vi "Write RC Parameters.vi"(0 "JSON FilePath":path=path "F:/Backup/ZenGage v3.0/20-02-2018/ZenGage v1.1/Configuration file/Rack Controller JSON/Rack Controller Override JSON.json", 1 "Part Name":string="102", 2 "RC parameters variant":variant, 5 "M and N array":T2(array[cluster])=[{"M1"=1, "M2"=2, "N1"=3, "N2"=4}, {"M1"=5, "M2"=6, "N1"=7, "N2"=8}, {"M1"=9, "M2"=10, "N1"=11, "N2"=12}], 7 "Enabled Disable Array":bool[](array[boolean]), 9 "Ticked measurements":i32[](array[numeric])=[0, 2, 4], 11 "error in (no error)":errorcluster, 12 "Rack Id":string="0", 13 "Variant":bool) -> (4 "JSON Variant":variant, 15 "error out":errorcluster)   [LabVIEW 2019, in "ZenGage v3.0 UI.lvclass"]
uses:
  ZenGage v3.0 UI.lvclass
panel:
  out "data":T1
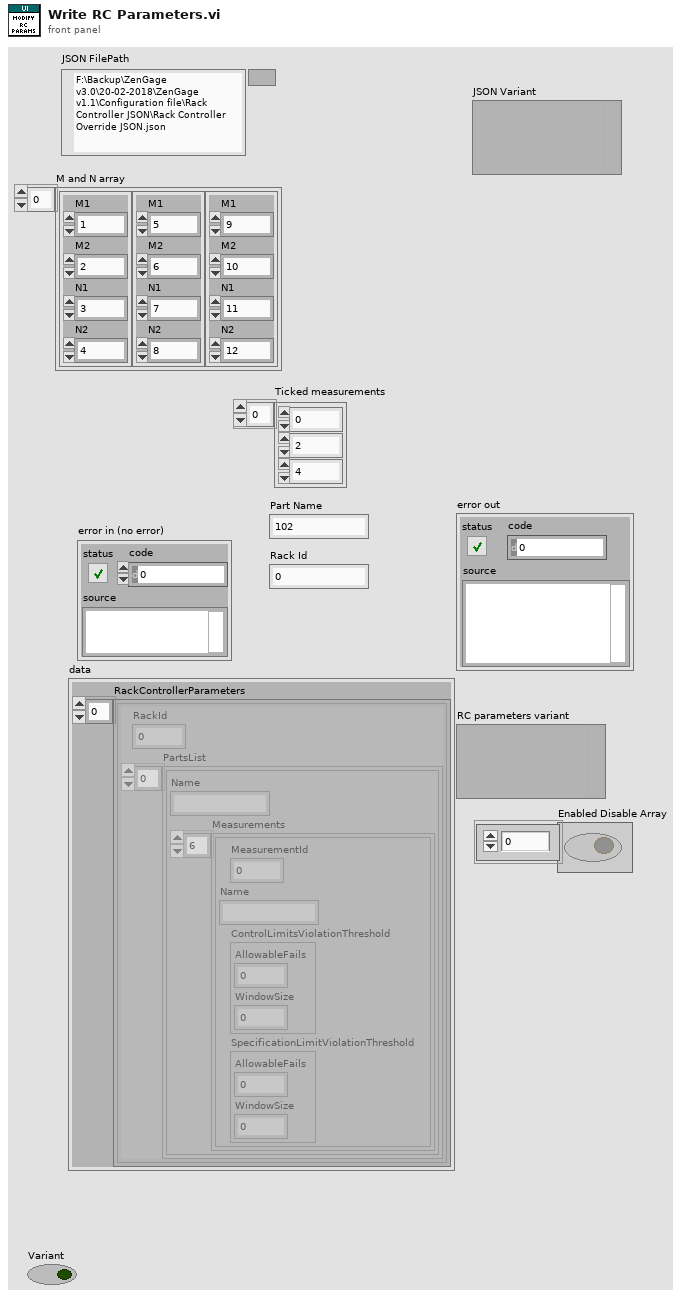
[diagram p1: front panel]
types:
  T1 = cluster{"RackControllerParameters":cluster{"RackId":dbl, "PartsList":cluster{"Name":string, "Measurements":cluster{"MeasurementId":dbl, "Name":string, "ControlLimitsViolationThreshold":cluster{"AllowableFails":dbl, "WindowSize":dbl}, "SpecificationLimitViolationThreshold":cluster{"AllowableFails":dbl, "WindowSize":dbl}}[]}[]}[]}
  T2 = cluster{"M1":u64, "M2":u64, "N1":u64, "N2":u64}[]
  T3 = enum16{"Action Failed", "Append", "Insert", "Replace"}
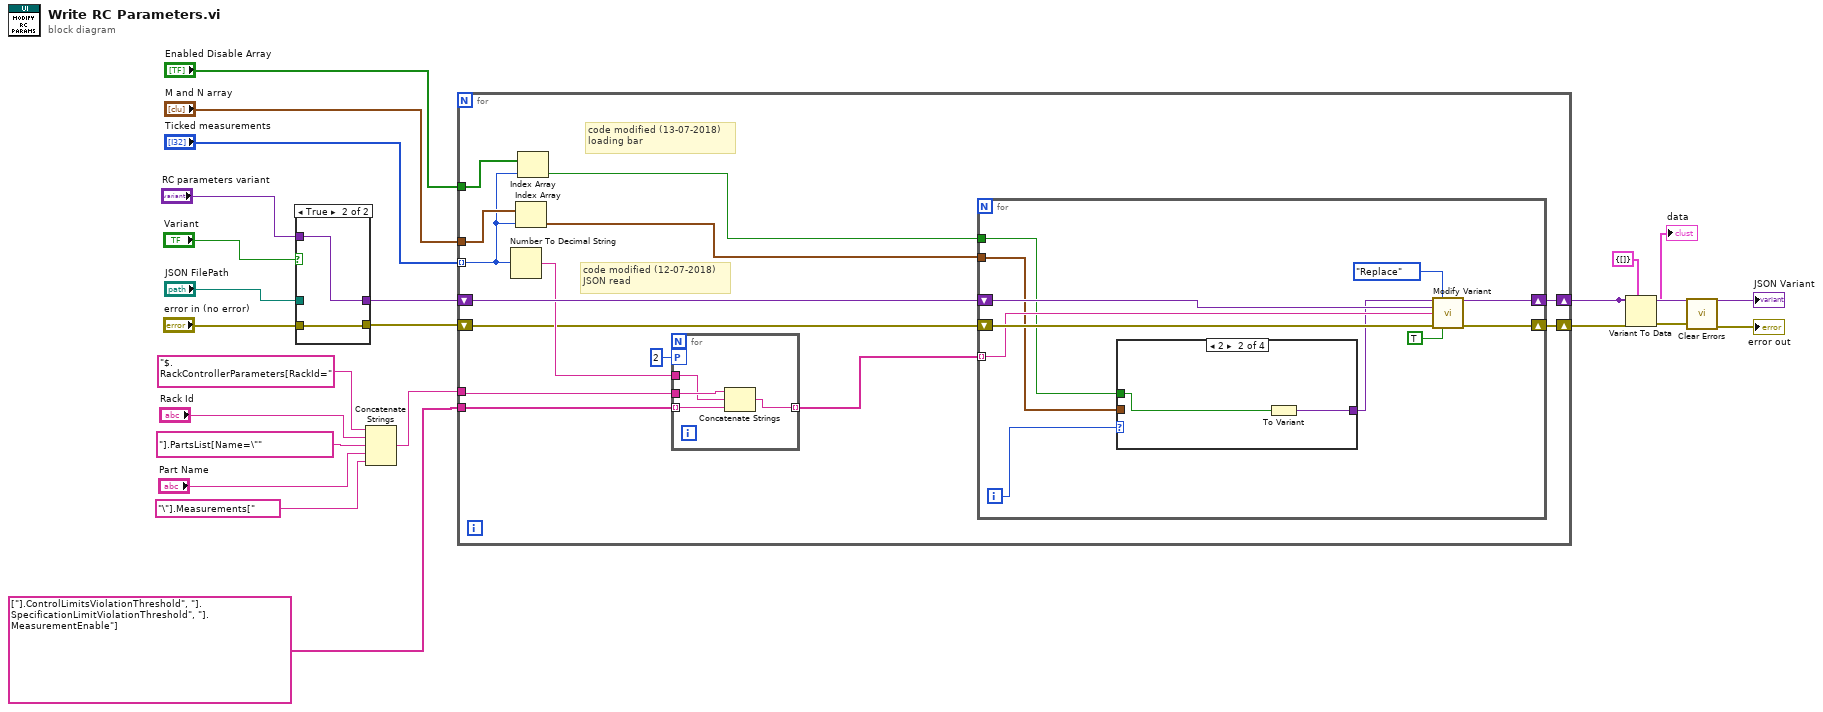
[diagram p0: block diagram]
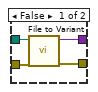
[diagram p2: hidden frame]
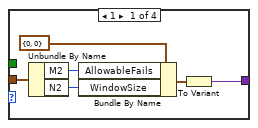
[diagram p3: hidden frame]
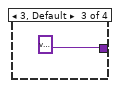
[diagram p4: hidden frame]
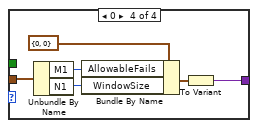
[diagram p5: hidden frame]
diagram:
  n1 = case shown="True" "Variant" {
    tunnel: "error in (no error)" -> [w26 w28]
    tunnel: [w25 w28] -> w19
    tunnel: "JSON FilePath" -> [w24 _]
    tunnel: [w23 w27] -> w17
    tunnel: "RC parameters variant" -> [_ w27]
    frame False {
      n2 = call <vilib>:"File to Variant.vi"("JSON FilePath"=w24, "error in (no error)"=w26) -> ("JSON Variant"=w23:variant, "error out"=w25:errorcluster)  [unwired: 6 in, 1 out]
    }
    frame True {
    }
  }
  n3 = Concatenate Strings("$.RackControllerParameters[RackId=", "Rack Id", "].PartsList[Name=\"", "Part Name", "\"].Measurements[") -> (w10:string)
  n4 = for {
    tunnel: "Ticked measurements" -> [w30] mode=indexing
    tunnel: "M and N array" -> [w35]
    shift-right: [w41] -> w7
    shift-left: w19 -> [w33]
    tunnel: w10 -> [w40]
    tunnel: string[] ["].ControlLimitsViolationThreshold", "].SpecificationLimitViolationThreshold", "].MeasurementEnable"] -> [w38]
    shift-right: [w36] -> w5
    shift-left: w17 -> [w42]
    tunnel: "Enabled Disable Array" -> [w31]
    # "code modified (13-07-2018)\nloading bar"
    # "code modified (12-07-2018)\nJSON read"
    n5 = Number To Decimal String(number=w30) -> (decimal integer string=w39:string)  [unwired: 1 in]
    n6 = Index Array(array=w35, index=w30) -> (element=w34:cluster{"M1":u64, "M2":u64, "N1":u64, "N2":u64})
    n7 = Index Array(array=w31, index=w30) -> (element=w29:bool)
    n8 = for {
      tunnel: w40 -> [w46]
      tunnel: w39 -> [w45]
      tunnel: w38 -> [w44] mode=indexing
      tunnel: [w43] -> w37 mode=indexing
      workers-P: 2 -> [_]
      n9 = Concatenate Strings(w46, w45, w44) -> (w43:string)
    }
    n10 = for {
      tunnel: w34 -> [w52]
      shift-right: [w55] -> w41
      shift-left: w33 -> [w57]
      tunnel: w37 -> [w54] mode=indexing
      shift-right: [w51] -> w36
      shift-left: w42 -> [w56]
      tunnel: w29 -> [w48]
      i -> [w49]
      n11 = case shown="2" w49 {
        tunnel: w52 -> [w63 _ _ w71]
        tunnel: [w59 w64 variant ("Variant") w68] -> w47
        tunnel: w48 -> [_ w65 _ _]
        frame 1 {
          n12 = Unbundle By Name(w63) -> ("M2"=w62:u64, "N2"=w61:u64)
          n13 = Bundle By Name(cluster=cluster{"AllowableFails":u64, "WindowSize":u64} {"AllowableFails"=0, "WindowSize"=0} ("ControlLimitsViolationThreshold"), "AllowableFails"=w62, "WindowSize"=w61) -> (w58:cluster{"AllowableFails":u64, "WindowSize":u64})
          n14 = To Variant(anything=w58) -> (Variant=w59:variant)
        }
        frame 2 {
          n15 = To Variant(anything=w65) -> (Variant=w64:variant)
        }
        frame 3, Default {
        }
        frame 0 {
          n16 = Unbundle By Name(w71) -> ("M1"=w70:u64, "N1"=w69:u64)
          n17 = Bundle By Name(cluster=cluster{"AllowableFails":u64, "WindowSize":u64} {"AllowableFails"=0, "WindowSize"=0} ("ControlLimitsViolationThreshold"), "AllowableFails"=w70, "WindowSize"=w69) -> (w67:cluster{"AllowableFails":u64, "WindowSize":u64})
          n18 = To Variant(anything=w67) -> (Variant=w68:variant)
        }
      }
      n19 = call <vilib>:"Modify Variant.vi"("New element in"=w47, "Functionality"=T3."Replace", "Parent variant in"=w56, "JSON query path"=w54, "error in (no error)"=w57, "Overwrite\n(Ignore datatype?)"=TRUE ("Overwrite\n(Ignore datatype?)")) -> ("VCluster out"=w51:variant, "error out"=w55:errorcluster)  [unwired: 5 in, 3 out]
    }
  }
  "JSON Variant" <- w5
  n20 = Variant To Data(error in=w7, type=T1 {"RackControllerParameters"=[]}, Variant=w5) -> (data=→"data":T1, error out=w6:errorcluster)
  n21 = call <vilib>:"Clear Errors.vi"("error in (no error)"=w6) -> ("error out"=→"error out":errorcluster)  [unwired: 5 in, 1 out]
